vi "Build Path.vi"(5 "Parallel in":refnum<class "Parallel.lvclass">, 6 "Path Builder":refnum<class "IPath Builder.lvclass">, 7 "Linked List ID":string, 8 "error in (no error)":errorcluster, 11 "Linked List Ref":refnum<data-value>) -> (0 "error out":errorcluster, 2 "Paths":path[](array[path]), 3 "Linked List Ref out":refnum<data-value>)   [LabVIEW 2017]
uses:
  888a9af0-6a9d-4290-98ca-e36b0c6a4dcd.vi
  Path Builder/IPath Builder/IPath Builder.lvclass
  data-type-serializer/source/String 1D/String 1D.lvclass
  C:/Users/jonmc/Documents/Git/Test Executive/gpm_packages/@cs/data-type-serializer/source/Data Type/Data Type.lvclass
  linked-list/Source/Linked List/ILinkedList/ILinked List.lvclass
  Parallel.lvclass
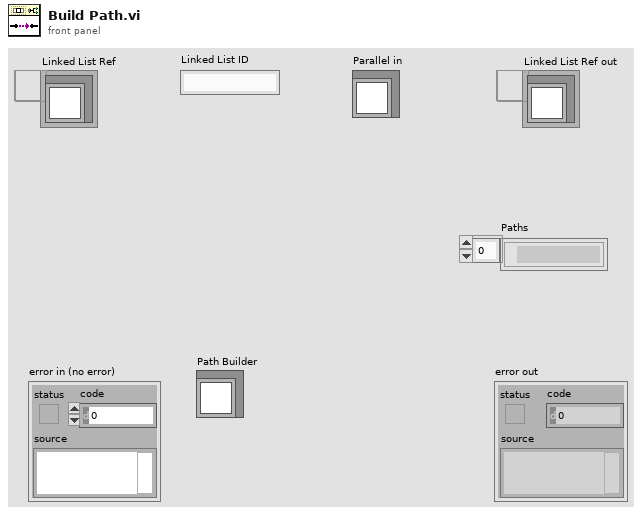
[diagram p1: front panel]
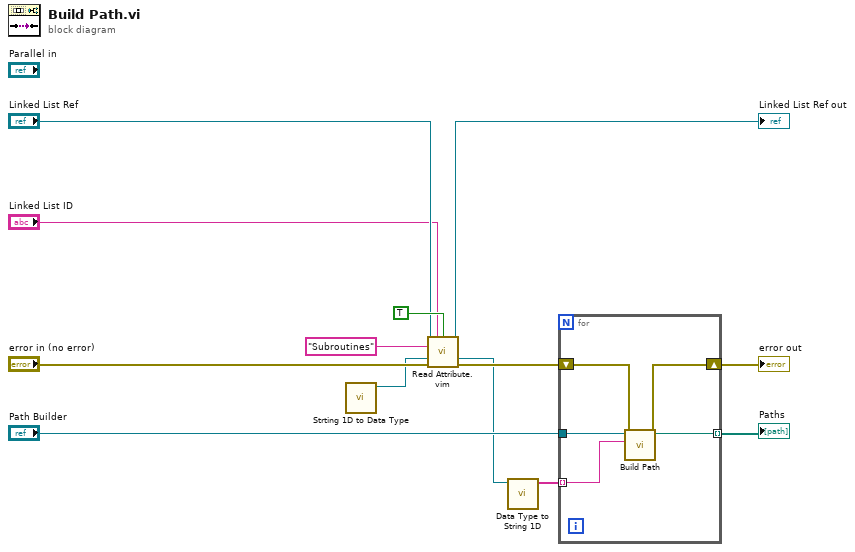
[diagram p0: block diagram]
diagram:
  n1 = call "Strting 1D to Data Type.vi"() -> ("Boolean out"=w4:refnum<class "String 1D.lvclass">)  [unwired: 10 in, 1 out]
  n2 = call "Read Attribute.vim"("Linked List Ref"="Linked List Ref", "Linked List ID"="Linked List ID", "Include Private?"=TRUE, "Attribute Name"="Subroutines", "Type"=w4, "error in (no error)"="error in (no error)") -> ("Linked List Ref out"=→"Linked List Ref out":refnum<data-value>, "Attribute"=w3:refnum<class "String 1D.lvclass">, "error out"=w11:errorcluster)  [unwired: 4 in, 3 out]
  n3 = call "Data Type to String 1D.vi"("Data Type"=w3) -> ("String 1D out"=w1:string[])  [unwired: 9 in, 1 out]
  n4 = for {
    tunnel: "Path Builder" -> [w17]
    tunnel: [w15] -> w2 mode=indexing
    shift-right: [w16] -> w5
    shift-left: w11 -> [w18]
    tunnel: w1 -> [w14] mode=indexing
    n5 = call-dynamic "Build Path.vi"("error in (no error)"=w18, "Path"=w14, "IPath Builder in"=w17) -> ("error out"=w16:errorcluster, "Path"=w15:path)  [unwired: 7 in]
  }
  "error out" <- w5
  "Paths" <- w2
